vi "toSequencedStringArray.vi"(8 "error in (no error)":errorcluster, 11 "ScriptEventList in":refnum<class "ScriptEventList.lvclass">) -> (0 "error out":errorcluster, 2 "Array":string[][](array[string]), 3 "ScriptEventList out":refnum<class "ScriptEventList.lvclass">)   [LabVIEW 2009, in "Tools.lvlib" / "Scripting.lvlib" / "ScriptEventList.lvclass"]
uses:
  ScriptEventList.lvclass
  ScriptEventList.lvclass/ScriptEventList.ctl
  ScriptEvent.lvclass
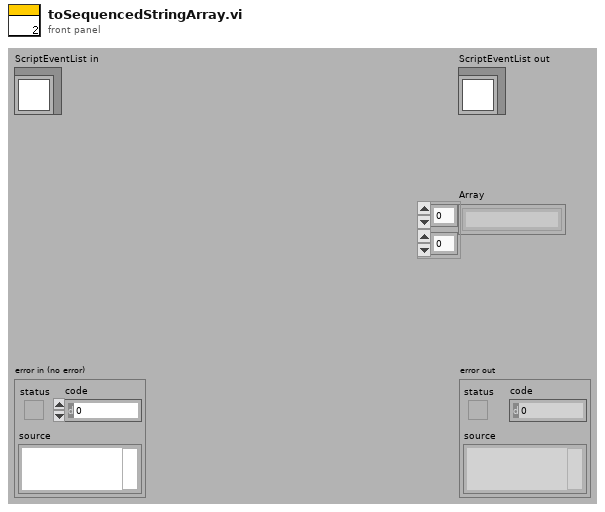
[diagram p1: front panel]
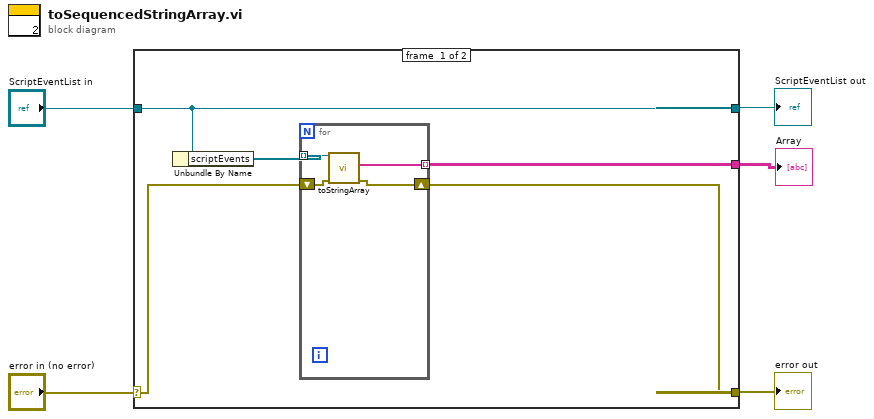
[diagram p0: block diagram]
diagram:
  n1 = case shown="No Error" "error in (no error)" {
    selector: "error in (no error)" -> [w8 w16]
    tunnel: [w7 w16] -> w4
    tunnel: [w10 w15] -> w2
    tunnel: "ScriptEventList in" -> [w10 w15]
    tunnel: [w6 _] -> w1
    frame #0 {
      n2 = Unbundle By Name(w10) -> ("scriptEvents"=w9:refnum<class "ScriptEvent.lvclass">[])
      n3 = for {
        tunnel: w9 -> [w13] mode=indexing
        shift-right: [w11] -> w7
        shift-left: w8 -> [w14]
        tunnel: [w12] -> w6 mode=indexing
        n4 = call-dynamic "toStringArray.vi"("error in (no error)"=w14, "ScriptEvent in"=w13) -> ("error out"=w11:errorcluster, "eventStringArray"=w12:string[])  [unwired: 7 in, 1 out]
      }
    }
    frame #1 {
    }
  }
  "error out" <- w4
  "ScriptEventList out" <- w2
  "Array" <- w1
